vi "Save Config.vi"(8 "error in (no error)":errorcluster, 9 "Config Format":T1, 10 "Path":path, 11 "VolatusConfig in":refnum<class "VolatusConfig.lvclass">) -> (0 "error out":errorcluster, 3 "VolatusConfig out":refnum<class "VolatusConfig.lvclass">)   [LabVIEW 2020, in "VolatusConfig.lvlib" / "VolatusConfig.lvclass"]
uses:
  VolatusConfig.lvclass
  Config Format.ctl
  VolatusConfig.lvclass/VolatusConfig.ctl
  lv-cdm/CDM-Config/Config-JSON/Config-JSON.lvclass
  C:/dev/lv20CE/relink/lv-cdm/CDM-Config/Config Storage/Config Storage.lvclass
  lv-cdm/CDM-Config/Config-INI/Config-INI.lvclass
  lv-cdm/CDM-Config/Config-Sqlite/Config-Sqlite.lvclass
  lv-cdm/CDM-Config/Config-JSON/Init.vi
  lv-cdm/CDM-Config/Config-INI/Init.vi
  lv-cdm/CDM-Config/Config-Sqlite/Init.vi
  VolatusConfig.lvlib
  lv-cdm/CDM-Config/Config Storage/Config Storage.lvclass
  Meta Name.ctl
  lv-cdm/CDM-Config/Config Element/Config Element.lvclass
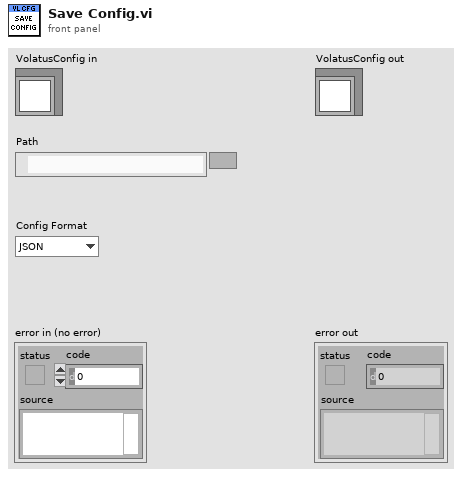
[diagram p1: front panel]
types:
  T1 = typedef "VolatusConfig.lvlib/Config Format.ctl" = enum16{"JSON", "INI", "SQLite"}
  T2 = typedef "VolatusConfig.lvlib/Meta Name.ctl" = enum16{"VL_Type", "VL_Node_IP", "VL_Node_Type", "VL_Task_Type", "VL_Group_Type", "VL_Channel_Type", "VL_Channel_DataType", "VL_Config_Version", "VL_Overlay_Type", "VL_Config_Hash"}
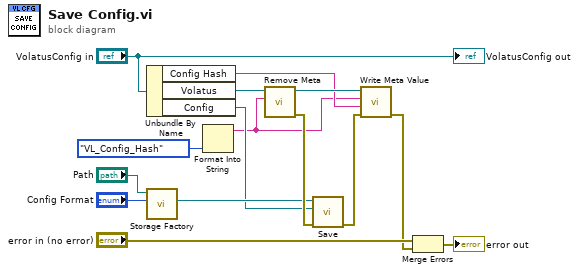
[diagram p0: block diagram]
diagram:
  n1 = Unbundle By Name("VolatusConfig in") -> ("Config Hash"=w4:string, "Volatus"=w7:refnum<class "Config Element.lvclass">, "Config"=w10:refnum<class "Config Manager.lvclass">)
  n2 = call "Storage Factory.vi"("Format"="Config Format", "Config Path"="Path") -> ("Storage"=w11:refnum<class "Config Storage.lvclass">)  [unwired: 9 in]
  n3 = Format Into String(Meta_Name."VL_Config_Hash" ("Meta Name")) -> (resulting string=w3:string)  [unwired: 3 in, 1 out]
  n4 = call "Remove Meta.vi"("Meta Name"=w3, "Config Element in"=w7) -> ("error out"=w15:errorcluster, "Config Element out"=w5:refnum<class "Config Element.lvclass">)  [unwired: 7 in, 1 out]
  n5 = call "Save.vi"("error in (no error)"=w15, "Config"=w10, "Config Storage in"=w11) -> ("error out"=w2:errorcluster)  [unwired: 7 in, 1 out]
  n6 = call "Write Meta Value.vi"("error in (no error)"=w2, "Meta Value"=w4, "Meta Name"=w3, "Config Element in"=w5) -> ("error out"=w1:errorcluster)  [unwired: 6 in, 1 out]
  n7 = Merge Errors("error in (no error)", w1) -> (→"error out":errorcluster)
  "VolatusConfig out" <- "VolatusConfig in"
